vi "Example application TCP.vi"() -> ()   [LabVIEW 2021, in "Example TCP.lvlib"]
uses:
  Example TCP.lvlib
  <vilib>/Platform/TimedLoop/XDataNode/timing_clust.ctl
  <vilib>/Platform/TimedLoop/XDataNode/nitl_modes.ctl
  <vilib>/Platform/TimedLoop/XDataNode/wakeup.ctl
  <vilib>/Platform/TimedLoop/XDataNode/XDataNode.xnode
  <vilib>/Platform/TimedLoop/XDataNode/XDNodeRunTimeDep.lvlib
panel:
  out "error out":errorcluster
  in  "save":bool
  out "read Temp":dbl
  in  "set Temp":dbl=100.0 format="%#_13g"
  in  "set GHI":dbl=100.0 format="%#_13g"
  in  "send sp":bool
  out "read GHI":dbl
  in  "stop":bool
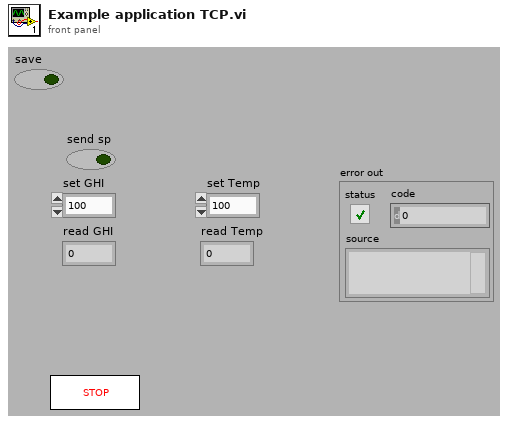
[diagram p1: front panel]
types:
  T1 = typedef "XDNodeRunTimeDep.lvlib/timing_clust.ctl" = cluster{"Expected End [f-1]":u64, "Actual End [f-1]":u64, "Finished Late? [f-1]":bool, "Expected End [i-1]":u64, "Actual End [i-1]":u64, "Finished Late? [i-1]":bool, "Expected Start [i]":u64, "Actual Start [i]":u64, "Expected Start [f]":u64, "Actual Start [f]":u64, "Source Name":string, "Structure Name":string, "Period":i64, "Deadline":i64, "Offset":i64, "Start":i64, "Priority":i32, "Timeout":i32, "Mode":T2, "Wakeup Reason":T3, "Error":errorcluster, "Source Type":string, "Secondary Source Type":string, "Global End Time":u64, "Global Start Time":u64, "Frame Duration":u64, "Iteration Duration":u64, "Assigned CPU":i32, "I/O Scan Engine Mode":u32}
  T2 = typedef "XDNodeRunTimeDep.lvlib/nitl_modes.ctl" = enum32{"No Change", "Process missed periods, maintain original phase", "Discard missed periods, maintain original phase", "Process missed periods, ignore original phase", "Discard missed periods, ignore original phase"}
  T3 = typedef "XDNodeRunTimeDep.lvlib/wakeup.ctl" = enum32{"Normal", "Aborted", "Asynchronous wakeup", "Timing source error", "Timed loop error", "Timeout"}
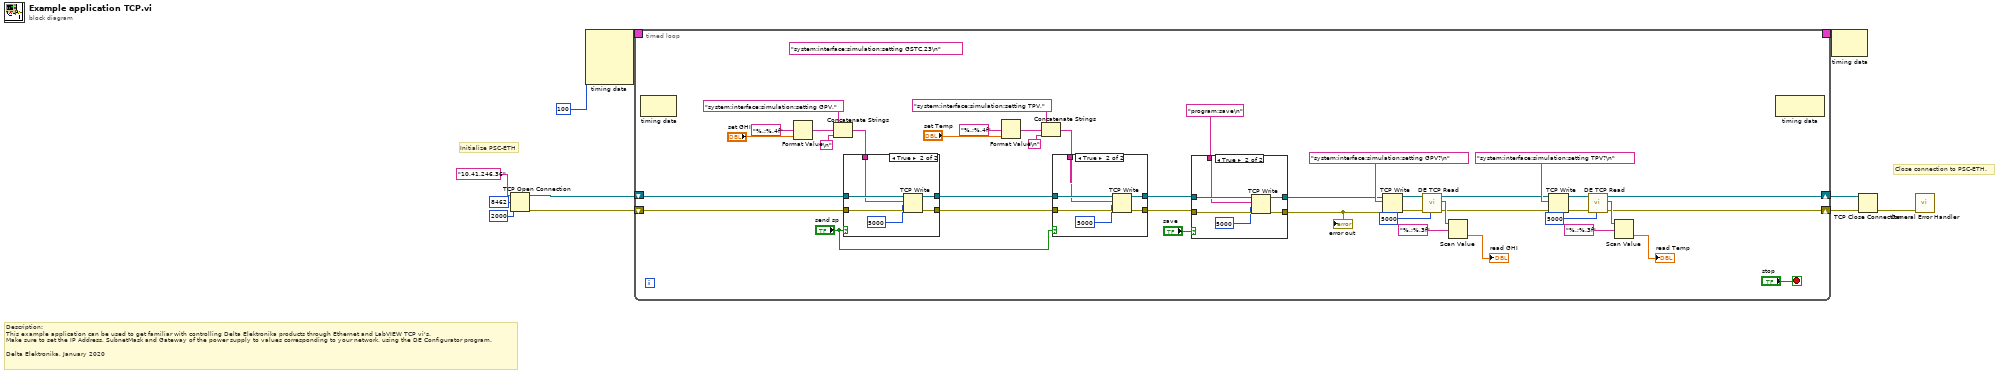
[diagram p0: block diagram]
diagram:
  # "Description:\nThis example application can be used to get familiar with controlling Delta Elektronika products through Ethernet and LabVIEW TCP vi's.\nMake sure to set the IP Address, SubnetMask and Gateway of the power supply to values corresponding to your network, using the DE Configurator program.\n\nDelta Elektronika, January 2020"
  # "Close connection to PSC-ETH."
  # "Initialize PSC-ETH"
  n1 = TCP Open Connection(address="10.41.246.36", remote port or service name=u16 8462 ("remote port"), timeout ms (60000)=2000) -> (connection ID=w5:refnum<k5>, error out=w4:errorcluster)  [unwired: 2 in]
  n2 = node-c288(i64 100 ("Period")) -> (w8:T1)  [unwired: 3 in]
  n3 = timed-loop {
    timing: w8 -> [_]
    timing-out: [_] -> w7
    shift-right: [w20] -> w2
    shift-left: w5 -> [w43]
    shift-right: [w19] -> w1
    shift-left: w4 -> [w42]
    stop <- "stop" stop-if-true
    (unwired) "system:interface:simulation:setting GSTC,23\n" ("data in")
    n4 = node-c288() -> ()  [unwired: 1 in, 1 out]
    n5 = Format Value(format string="%.;%.4f", value (0)="set GHI") -> (output string=w53:string)  [unwired: 1 in]
    n6 = Concatenate Strings("system:interface:simulation:setting GPV," ("data in"), w53, "\n" ("string")) -> (w40:string)
    n7 = case shown="True" "send sp" {
      tunnel: w42 -> [w72 w79]
      tunnel: w43 -> [w73 w78]
      tunnel: w40 -> [_ w77]
      tunnel: [w73 w76] -> w32
      tunnel: [w72 w75] -> w31
      frame False {
      }
      frame True {
        n8 = TCP Write(connection ID=w78, data in=w77, error in (no error)=w79, 9:5000 ("timeout ms (25000)")) -> (connection ID out=w76:refnum<k5>, error out=w75:errorcluster)  [unwired: 1 out]
      }
    }
    n9 = Format Value(format string="%.;%.4f", value (0)="set Temp") -> (output string=w39:string)  [unwired: 1 in]
    n10 = Concatenate Strings("system:interface:simulation:setting TPV," ("data in"), w39, "\n" ("string")) -> (w34:string)
    n11 = case shown="True" "send sp" {
      tunnel: w31 -> [w62 w69]
      tunnel: w32 -> [w63 w68]
      tunnel: w34 -> [_ w67]
      tunnel: [w63 w66] -> w18
      tunnel: [w62 w65] -> w17
      frame False {
      }
      frame True {
        n12 = TCP Write(connection ID=w68, data in=w67, error in (no error)=w69, 9:5000 ("timeout ms (25000)")) -> (connection ID out=w66:refnum<k5>, error out=w65:errorcluster)  [unwired: 1 out]
      }
    }
    n13 = case shown="True" "save" {
      tunnel: w17 -> [w54 w61]
      tunnel: w18 -> [w55 w60]
      tunnel: "program:save\n" ("data in") -> [_ w59]
      tunnel: [w55 w58] -> w15
      tunnel: [w54 w57] -> w14
      frame False {
      }
      frame True {
        n14 = TCP Write(connection ID=w60, data in=w59, error in (no error)=w61, 9:5000 ("timeout ms (25000)")) -> (connection ID out=w58:refnum<k5>, error out=w57:errorcluster)  [unwired: 1 out]
      }
    }
    "error out" <- w14
    n15 = TCP Write(connection ID=w15, data in="system:interface:simulation:setting GPV?\n", error in (no error)=w14) -> (connection ID out=w48:refnum<k5>, error out=w47:errorcluster)  [unwired: 1 in, 1 out]
    n16 = call "DE TCP Read.vi"("timeout ms (25000)"=5000, "error in (no error)"=w47, "Connection ID in"=w48) -> ("error out"=w23:errorcluster, "TCP Read data"=w46:string, "Connection ID out"=w24:refnum<k5>)  [unwired: 6 in]
    n17 = Scan Value(string=w46, format string="%.;%.3f") -> (value=→"read GHI":dbl)  [unwired: 1 in, 1 out]
    n18 = TCP Write(connection ID=w24, data in="system:interface:simulation:setting TPV?\n", error in (no error)=w23) -> (connection ID out=w29:refnum<k5>, error out=w28:errorcluster)  [unwired: 1 in, 1 out]
    n19 = call "DE TCP Read.vi"("timeout ms (25000)"=5000, "error in (no error)"=w28, "Connection ID in"=w29) -> ("error out"=w19:errorcluster, "TCP Read data"=w27:string, "Connection ID out"=w20:refnum<k5>)  [unwired: 6 in]
    n20 = Scan Value(string=w27, format string="%.;%.3f") -> (value=→"read Temp":dbl)  [unwired: 1 in, 1 out]
    n21 = node-c288() -> ()  [unwired: 1 in, 1 out]
  }
  n22 = node-c288(w7) -> ()  [unwired: 1 out]
  n23 = TCP Close Connection(connection ID=w2, error in (no error)=w1) -> (error out=w3:errorcluster)  [unwired: 1 in, 1 out]
  n24 = call <vilib>:"General Error Handler.vi"("error in (no error)"=w3) -> ()  [unwired: 10 in, 5 out]
